vi "Rectangle.vi"(4 "Properties":T1={"Color"=2147483647, "Line"={"Style"=enum."Automatic", "Color"=2147483647, "Width"=nan}, "Display"={"Alpha"=nan, "Z Order"=nan}} {"Color" items=["Automatic"=2147483647, "Black"=0, "White"=16777215, "Red"=16711680, "Green"=2263842, "Blue"=255, "Cyan"=65535, "Magenta"=16711935, "Yellow"=16776960]; "Line"."Color" items=["Automatic"=2147483647, "Black"=0, "White"=16777215, "Red"=16711680, "Green"=2263842, "Blue"=255, "Cyan"=65535, "Magenta"=16711935, "Yellow"=16776960]}, 5 "Height":dbl, 7 "Width":dbl, 8 "error in (no error)":errorcluster, 9 "Y Position":dbl, 10 "X Position":dbl, 11 "Plot ID":T6 format="%x") -> (0 "error out":errorcluster, 3 "Plot ID Out":T6 format="%x")   [LabVIEW 2013, in "Advanced Plotting Toolkit.lvlib"]
doc: "Draw a rectangle on the plot, in data coordinates."
uses:
  Advanced Plotting Toolkit.lvlib
  typedefs/PlotID.ctl
  ShapeProperties.ctl
  typedefs/PlotColor.ctl
  properties/Line.ctl
  properties/Line_Style.ctl
  properties/Display.ctl
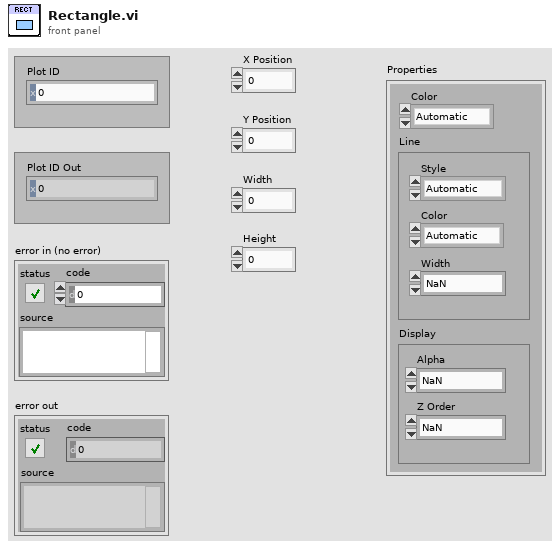
[diagram p1: front panel]
types:
  T1 = typedef "Advanced Plotting Toolkit.lvlib/ShapeProperties.ctl" = cluster{"Color":T2, "Line":T3, "Display":T5}
  T2 = typedef "Advanced Plotting Toolkit.lvlib/PlotColor.ctl" = u32
  T3 = typedef "Advanced Plotting Toolkit.lvlib/Line.ctl" = cluster{"Style":T4, "Color":T2, "Width":sgl}
  T4 = typedef "Advanced Plotting Toolkit.lvlib/Line_Style.ctl" = enum16{"Automatic", "Solid", "Dashed", "Dotted", "Dash-dot", "Invisible"}
  T5 = typedef "Advanced Plotting Toolkit.lvlib/Display.ctl" = cluster{"Alpha":dbl, "Z Order":dbl}
  T6 = typedef "Advanced Plotting Toolkit.lvlib/PlotID.ctl" = i32
  T7 = typedef "Advanced Plotting Toolkit.lvlib/KeyValue.ctl" = cluster{"Key":string, "Value":string}
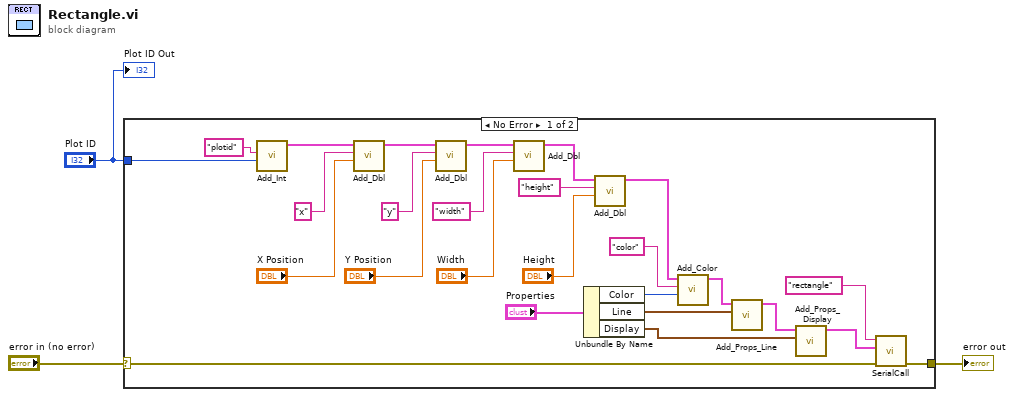
[diagram p0: block diagram]
diagram:
  n1 = case shown="No Error" "error in (no error)" {
    selector: "error in (no error)" -> [w28 w30]
    tunnel: "Plot ID" -> [w29 _]
    tunnel: [w27 w30] -> w1
    frame No Error {
      n2 = call "Add_Int.vi"("Value"=w29, "Key"="plotid") -> ("Keyword Array Out"=w18:T7[])  [unwired: 9 in]
      n3 = call "Add_Dbl.vi"("Value"="X Position", "Key"="x", "Keyword Array"=w18) -> ("Keyword Array Out"=w17:T7[])  [unwired: 8 in]
      n4 = call "Add_Dbl.vi"("Value"="Y Position", "Key"="y", "Keyword Array"=w17) -> ("Keyword Array Out"=w16:T7[])  [unwired: 8 in]
      n5 = call "Add_Dbl.vi"("Value"="Width", "Key"="width", "Keyword Array"=w16) -> ("Keyword Array Out"=w5:T7[])  [unwired: 8 in]
      n6 = Unbundle By Name("Properties") -> ("Color"=w14:T2, "Line"=w12:T3, "Display"=w11:T5)
      n7 = call "Add_Dbl.vi"("Value"="Height", "Key"="height", "Keyword Array"=w5) -> ("Keyword Array Out"=w4:T7[])  [unwired: 8 in]
      n8 = call "Add_Color.vi"("Color"=w14, "Key"="color", "Keyword Array"=w4) -> ("Keyword Array Out"=w10:T7[])  [unwired: 8 in]
      n9 = call "Add_Props_Line.vi"("Line"=w12, "Keyword Array"=w10) -> ("Keyword Array Out"=w9:T7[])  [unwired: 9 in]
      n10 = call "Add_Props_Display.vi"("Display"=w11, "Keyword Array"=w9) -> ("Keyword Array Out"=w8:T7[])  [unwired: 9 in]
      n11 = call "SerialCall.vi"("error in (no error)"=w28, "data"=w8, "Resource"="rectangle") -> ("error out"=w27:errorcluster)  [unwired: 7 in, 1 out]
    }
    frame Error {
    }
  }
  "error out" <- w1
  "Plot ID Out" <- "Plot ID"
